vi "Initialize_New_Sets_of_Tracks-1.vi"(4 "[IN] # of Eleme\nnts in New Tracks":i32, 5 "[IN] # previously \nconnected tracks":i32) -> (1 "[OUT] Clusters for Re\nconstructed Tracks":T1)   [LabVIEW 2013]
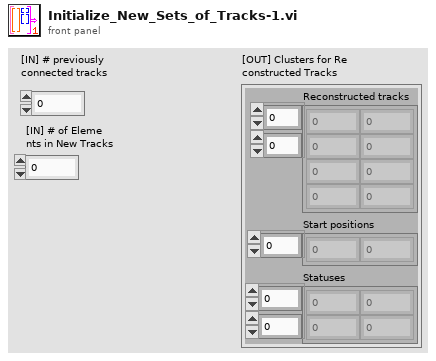
[diagram p1: front panel]
types:
  T1 = cluster{"Reconstructed tracks":dbl[][], "Start positions":i32[], "Statuses":i16[][]}
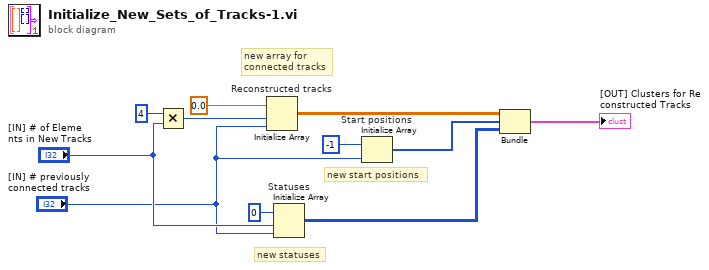
[diagram p0: block diagram]
diagram:
  # "new statuses"
  # "new start positions"
  # "new array for \nconnected tracks"
  n1 = Multiply(x=4, y="[IN] # of Eleme\nnts in New Tracks") -> (x*y=w9:i32)
  n2 = Initialize Array "Reconstructed tracks"(0.0 ("element"), w9, "[IN] # previously \nconnected tracks") -> (w4:dbl[][])
  n3 = Initialize Array "Statuses"(i16 0 ("element"), "[IN] # of Eleme\nnts in New Tracks", "[IN] # previously \nconnected tracks") -> (w2:i16[][])
  n4 = Initialize Array "Start positions"(-1 ("x"), "[IN] # previously \nconnected tracks") -> (w3:i32[])
  n5 = Bundle(w4, w3, w2) -> (→"[OUT] Clusters for Re\nconstructed Tracks":cluster{dbl[][], i32[], i16[][]})  [unwired: 1 in]
